vi "2. Show MassDataa Cache Status in FP.vi"() -> ()   [LabVIEW 2017]
uses:
  MassData-Parameter/Utility/Def-MassData Status Indicator(Vertical).ctl
  MassData-Parameter/Utility/Def-MassData Status Indicator(Horizontal).ctl
  9f0fb4c0-febd-4984-af95-02e44bfd84b8.vi
  51626e05-d687-430a-8a18-306667d64ebb.vi
  MassData-Parameter/_support/FGV-MassData.vi
  MassData-Parameter/CSM MassData Parameter Support.lvlib
panel:
  out "MassData Status Horizontal":T1={"w"={287840.0, 276144.0}, "r"={287840.0, 276144.0}} {"r" scale=1.0..5000000.0 scale format="%#_6p"; "w" scale=1.0..5000000.0 scale format="%#_6p"}
  in  "stop":bool
  out "MassData Status Vertical":T2={"w"={287840.0, 276144.0}, "r"={287840.0, 276144.0}} {"r" scale=1.0..5000000.0 scale format="%#_6p"; "w" scale=1.0..5000000.0 scale format="%#_6p"}
  out "Argument":string
  out "Waveform Graph":waveform(dbl)(graph)
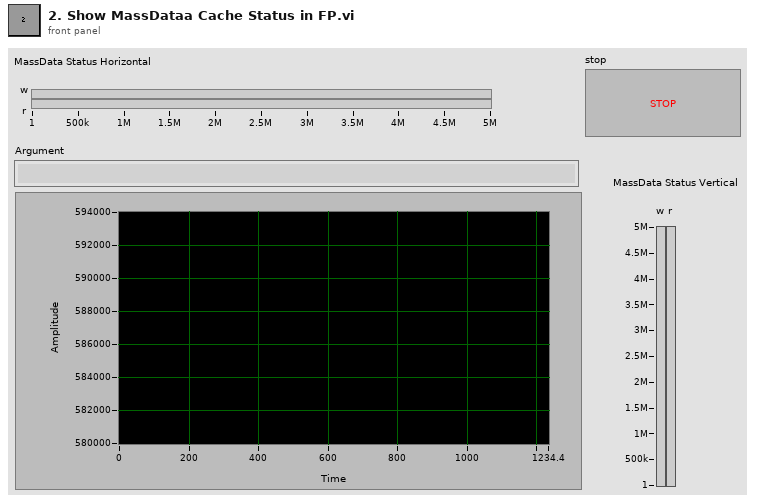
[diagram p1: front panel]
types:
  T1 = typedef "Def-MassData Status Indicator(Horizontal).ctl" = cluster{"w":cluster{dbl, dbl}, "r":cluster{dbl, dbl}}
  T2 = typedef "Def-MassData Status Indicator(Vertical).ctl" = cluster{"w":cluster{dbl, dbl}, "r":cluster{dbl, dbl}}
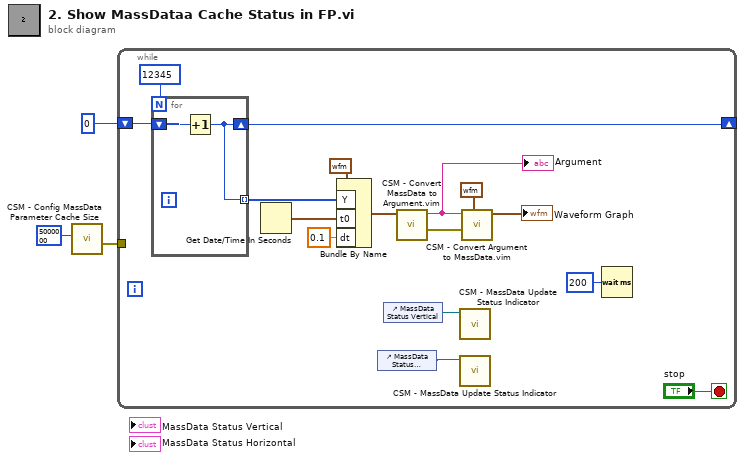
[diagram p0: block diagram]
diagram:
  n1 = call "CSM - Config MassData Parameter Cache Size.vi"("size(1M)"=5000000) -> ("Error out"=w1:errorcluster)  [unwired: 10 in]
  n2 = while {
    shift-right: [w15] -> _
    shift-left: 0 -> [w16]
    tunnel: w1 -> [_]
    stop <- "stop" stop-if-true
    n3 = for {
      N: 12345 -> [_]
      tunnel: [w20] -> w11 mode=indexing
      shift-right: [w20] -> w15
      shift-left: w16 -> [w21]
      n4 = Increment(x=w21) -> (x+1=w20:i32)
    }
    n5 = Get Date/Time In Seconds() -> (seconds since 1Jan1904=w13:timestamp)
    n6 = Bundle By Name(cluster=waveform(dbl) {"t0"=timestamp(0 s since 1904-01-01), "dt"=1.0, "Y"=[]} ("Waveform"), "Y"=w11, "t0"=w13, "dt"=0.1) -> (w9:waveform(dbl))
    n7 = control-ref of="MassData Status Horizontal"() -> (w5:refnum<vi>)
    n8 = control-ref of="MassData Status Vertical"() -> (w6:refnum<vi>)
    n9 = call "CSM - Convert MassData to Argument.vim"("DBL"=w9) -> ("error out"=w7:errorcluster, "MassData Argument"=w8:string)  [unwired: 7 in]
    "Argument" <- w8
    n10 = call "CSM - MassData Update Status Indicator.vi"("MassData Status Indicator"=w6) -> ()  [unwired: 10 in, 1 out]
    n11 = call "CSM - MassData Update Status Indicator.vi"("MassData Status Indicator"=w5) -> ()  [unwired: 10 in, 1 out]
    n12 = call "CSM - Convert Argument to MassData.vim"("Type"=waveform(dbl) {"t0"=timestamp(0 s since 1904-01-01), "dt"=1.0, "Y"=[]} ("output waveform"), "error in (no error)"=w7, "MassData Argument"=w8) -> ("Data"=→"Waveform Graph":waveform(dbl))  [unwired: 5 in, 1 out]
    n13 = Wait (ms)(milliseconds to wait=u32 200) -> ()  [unwired: 1 out]
  }
